vi "212format_work_Init.vi"(0 "object in":refnum<class "212format_work.lvclass">, 5 "error in (no error)":errorcluster) -> (14 "object out":refnum<class "212format_work.lvclass">, 19 "error out":errorcluster)   [LabVIEW 2016, in "212format_work.lvclass"]
uses:
  212format_work.lvclass
  interface_class/interface.lvclass
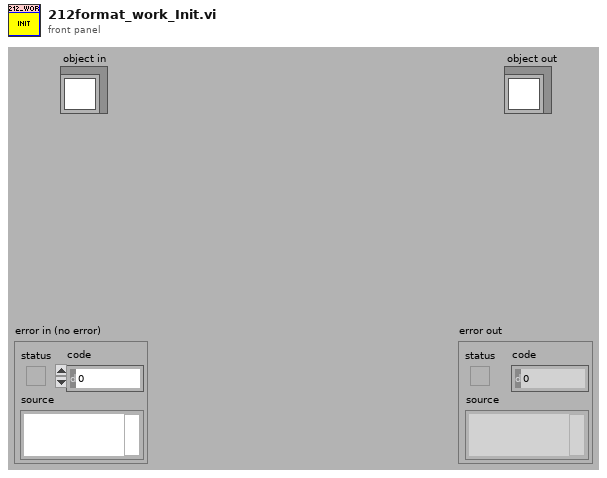
[diagram p1: front panel]
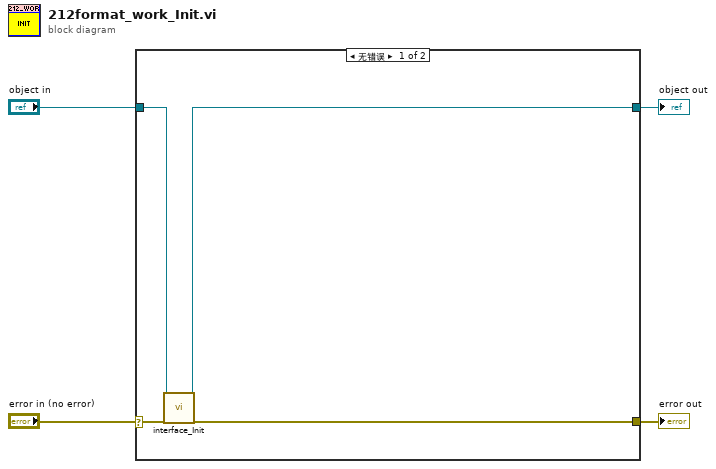
[diagram p0: block diagram]
diagram:
  n1 = case shown="无错误" "error in (no error)" {
    selector: "error in (no error)" -> [w8 w9]
    tunnel: [w5 w10] -> w4
    tunnel: "object in" -> [w6 w10]
    tunnel: [w7 w9] -> w1
    frame No Error {
      n2 = call "interface_Init.vi"("object in"=w6, "error in (no error)"=w8) -> ("object out"=w5:refnum<class "212format_work.lvclass">, "error out"=w7:errorcluster)  [unwired: 15 in, 1 out]
    }
    frame Error {
    }
  }
  "object out" <- w4
  "error out" <- w1
